vi "Op Point Linear Interpolation.vi"(8 "error in (no error)":errorcluster, 11 "BaseProducer in":refnum<class "BaseProducer.lvclass">) -> (0 "error out":errorcluster, 3 "BaseProducer out":refnum<class "BaseProducer.lvclass">)   [LabVIEW 2013, in "BaseProducer.lvclass"]
doc: "This method linearly interpolates between the current state and the next desired state, determining rates of change for each state, and a time target for the command loop. The rate of change is pegged at a maximum for the state that has to go the furthest, and the other rates are calculated based on the associated time target.\n\nNow it also creates an array of step-wise states between the current state and the target state. It either creates a specified number of steps, or however many steps are needed to get to the target state using a minimum step size, whichever results in fewer steps."
uses:
  BaseProducer.lvclass
  BaseProducer.lvclass/BaseProducer.ctl
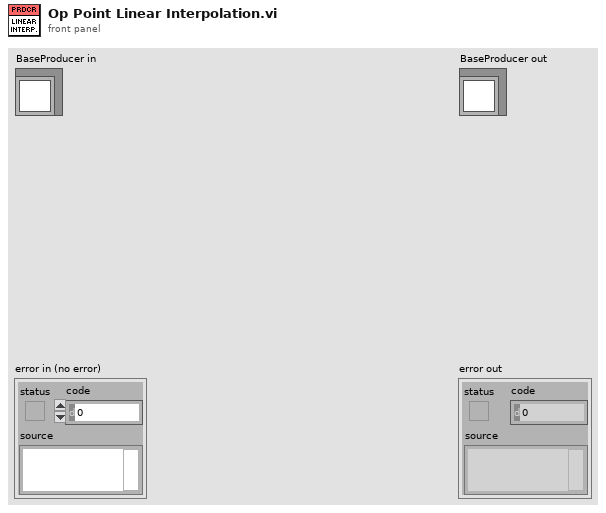
[diagram p1: front panel]
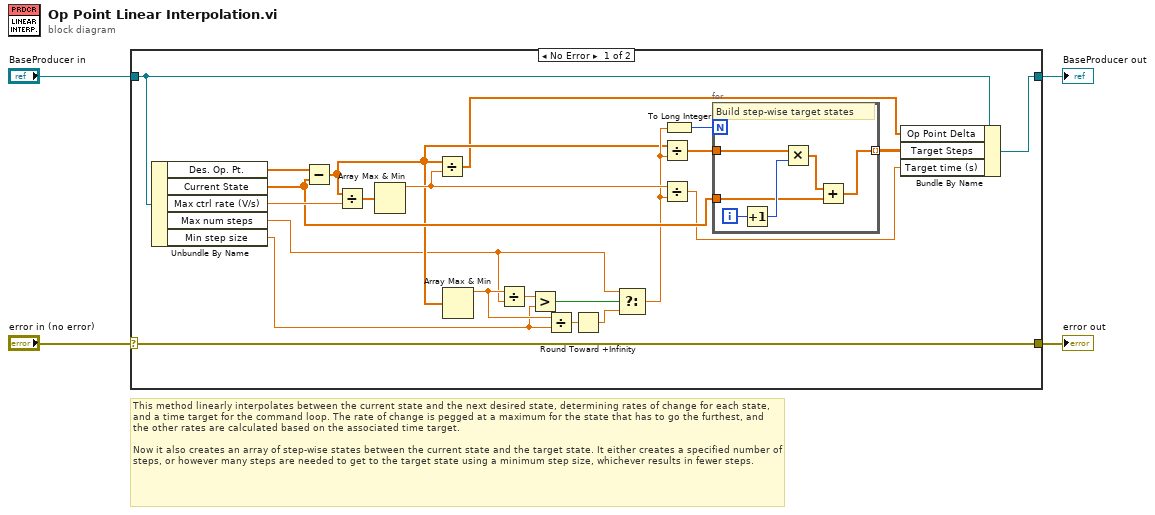
[diagram p0: block diagram]
diagram:
  # "This method linearly interpolates between the current state and the next desired state, determining rates of change for each state, and a time target for the command loop. The rate of change is pegged at a maximum for the state that has to go the furthest, and the other rates are calculated based on the associated time target.\n\nNow it also creates an array of step-wise states between the current state and the target state. It either creates a specified number of steps, or however many steps are needed to get to the target state using a minimum step size, whichever results in fewer steps."
  n1 = case shown="No Error" "error in (no error)" {
    selector: "error in (no error)" -> [w26 w34]
    tunnel: [w26 w34] -> w3
    tunnel: [w21 w33] -> w1
    tunnel: "BaseProducer in" -> [w22 w33]
    frame No Error {
      n2 = Unbundle By Name(w22) -> ("Des. Op. Pt."=w25:dbl[], "Current State"=w15:dbl[], "Max ctrl rate (V/s)"=w24:dbl, "Max num steps"=w7:dbl, "Min step size"=w6:dbl)
      n3 = Subtract(x=w25, y=w15) -> (x-y=w10:dbl[])
      n4 = Divide(x=w10, y=w24) -> (x/y=w23:dbl[])
      n5 = Array Max & Min(array=w23) -> (max value=w14:dbl)  [unwired: 3 out]
      n6 = Divide(x=w10, y=w14) -> (x/y=w8:dbl[])
      n7 = Array Max & Min(array=w10) -> (max value=w18:dbl)  [unwired: 3 out]
      n8 = Divide(x=w18, y=w7) -> (x/y=w20:dbl)
      n9 = Greater?(x=w20, y=w6) -> (0:w19:bool)
      n10 = Divide(x=w18, y=w6) -> (x/y=w17:dbl)
      n11 = Round Toward +Infinity(x=w17) -> (ceil(x): smallest int >= x=w9:dbl)
      n12 = Select(t=w7, s=w19, f=w9) -> (s? t:f=w12:dbl)
      n13 = Divide(x=w10, y=w12) -> (x/y=w11:dbl[])
      n14 = Divide(x=w14, y=w12) -> (x/y=w13:dbl)
      n15 = To Long Integer(number=w12) -> (32bit integer=w16:i32)
      n16 = for {
        N: w16 -> [_]
        tunnel: w11 -> [w27]
        tunnel: w15 -> [w30]
        tunnel: [w29] -> w5 mode=indexing
        i -> [w32]
        # "Build step-wise target states"
        n17 = Increment(x=w32) -> (x+1=w31:i32)
        n18 = Multiply(x=w27, y=w31) -> (x*y=w28:dbl[])
        n19 = Add(x=w28, y=w30) -> (x+y=w29:dbl[])
      }
      n20 = Bundle By Name(cluster=w22, "Op Point Delta"=w8, "Target Steps"=w5, "Target time (s)"=w13) -> (w21:refnum<class "BaseProducer.lvclass">)
    }
    frame Error {
    }
  }
  "error out" <- w3
  "BaseProducer out" <- w1
